vi "Worker Name & Path.vi"(10 "Variant":string, 11 "Worker":string) -> (0 "error out":errorcluster, 1 "Is Worker Variant":bool, 2 "lvlib Path":path, 3 "Display Name":string, 5 "Icon":T1)   [LabVIEW 2022 SP3, in "FlexBlocks Support.lvlib"]
uses:
  FlexBlocks Support.lvlib
  <vilib>/picture/picture.llb/imagedata.ctl
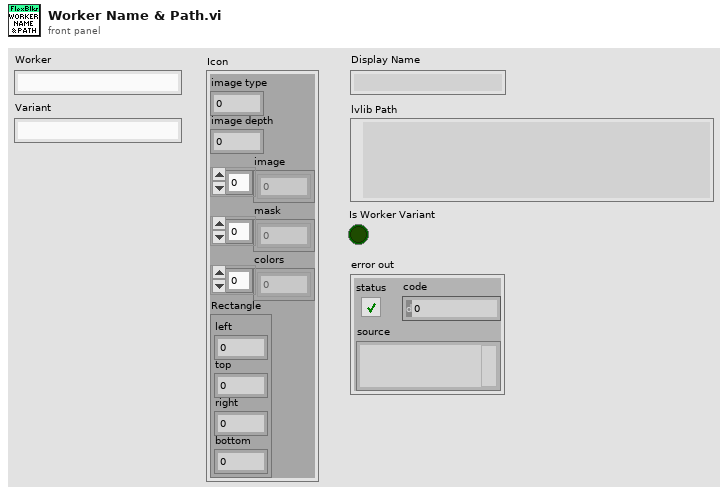
[diagram p1: front panel]
types:
  T1 = typedef "imagedata.ctl" = cluster{"image type":i32, "image depth":i32, "image":u8[], "mask":u8[], "colors":u32[], "Rectangle":cluster{"left":i16, "top":i16, "right":i16, "bottom":i16}}
  T2 = typedef "FlexBlocks Support.lvlib/Paths.ctl" = cluster{"FlexBlocks":path, "Workers Root":path, "Specialized Editors":path, "Worker Template":path, "SM Template":path, "Read Control Value Vim":path, "Write Indicator Value Vim":path}
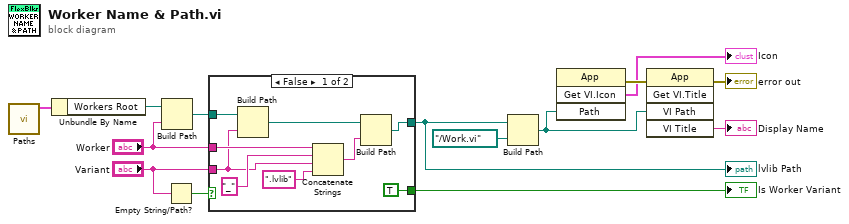
[diagram p0: block diagram]
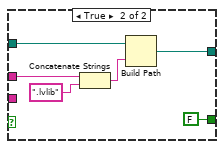
[diagram p2: hidden frame]
diagram:
  n1 = call "Paths.vi"() -> ("Paths"=w5:T2)  [unwired: 11 in]
  n2 = Unbundle By Name(w5) -> ("Workers Root"=w4:path)
  n3 = Build Path(base path=w4, name or relative path="Worker") -> (appended path=w11:path)
  n4 = Empty String/Path?(string/path="Variant") -> (empty?=w14:bool)
  n5 = case shown="False" w14 {
    tunnel: "Variant" -> [w20 _]
    tunnel: "Worker" -> [w23 w29]
    tunnel: w11 -> [w21 w27]
    tunnel: [w16 w25] -> w7
    tunnel: [TRUE FALSE] -> w8
    frame False {
      n6 = Build Path(base path=w21, name or relative path=w20) -> (appended path=w18:path)
      n7 = Concatenate Strings(w23, "_" ("string"), w20, ".lvlib" ("string")) -> (w17:string)
      n8 = Build Path(base path=w18, name or relative path=w17) -> (appended path=w16:path)
    }
    frame True {
      n9 = Concatenate Strings(w29, ".lvlib" ("string")) -> (w26:string)
      n10 = Build Path(base path=w27, name or relative path=w26) -> (appended path=w25:path)
    }
  }
  "lvlib Path" <- w7
  "Is Worker Variant" <- w8
  n11 = Build Path(base path=w7, name or relative path=path "../Work.vi") -> (appended path=w1:path)
  n12 = invoke class="App" method="Get VI.Icon"("Path"=w1) -> (error out=w3:errorcluster, "Get VI.Icon"=→"Icon":T1)  [unwired: 3 in, 2 out]
  n13 = invoke class="App" method="Get VI.Title"(error in=w3, "VI Path"=w1) -> (error out=→"error out":errorcluster, "VI Title"=→"Display Name":string)  [unwired: 3 in, 3 out]
